vi "change channel raw default value.vi"(7 "owner ID":string, 8 "error in":errorcluster, 9 "raw default":string, 10 "channel name":string, 11 "engine configuration in":refnum<class "base TBM sequencer configuration.lvclass">) -> (0 "error out":errorcluster, 3 "engine configuration out":refnum<class "base TBM sequencer configuration.lvclass">)   [LabVIEW 2014, in "base TBM sequencer configuration.lvclass"]
uses:
  base TBM sequencer configuration.lvclass
  <vilib>/NI/Tag Bus/tag/tag descriptor.lvclass
  <vilib>/NI/Tag Bus/tag/tag descriptor.lvclass/tag descriptor.ctl
  base TBM sequencer configuration.lvclass/base TBM sequencer configuration.ctl
  <vilib>/NI/Tag Bus/tag/write tag name.vi
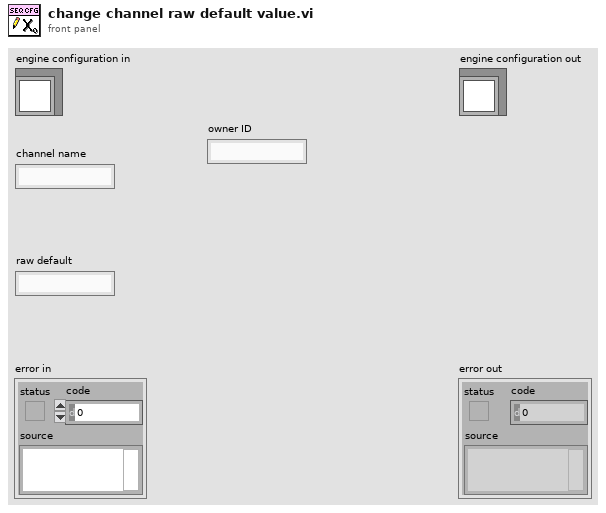
[diagram p1: front panel]
types:
  T1 = typedef "base TBM sequencer configuration.lvclass/Tag Info.ctl" = cluster{"Channel":refnum<class "TBM channel.lvclass">, "Writers":string[], "Readers":string[], "Owning ID":string}
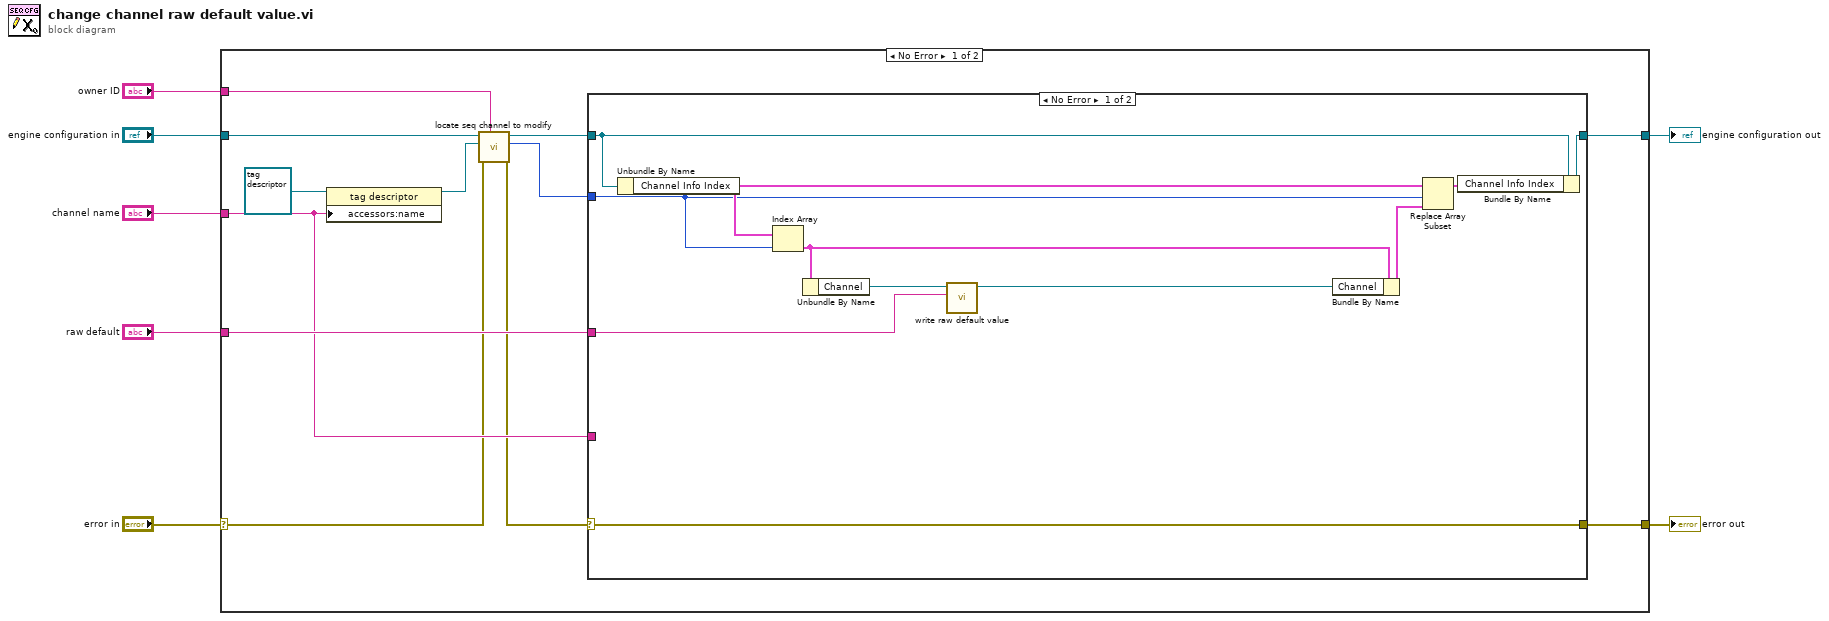
[diagram p0: block diagram]
diagram:
  n1 = case shown="No Error" "error in" {
    selector: "error in" -> [w10 w34]
    tunnel: [w17 w34] -> w6
    tunnel: [w18 w33] -> w4
    tunnel: "engine configuration in" -> [w14 w33]
    tunnel: "channel name" -> [w15 _]
    tunnel: "raw default" -> [w16 _]
    tunnel: "owner ID" -> [w11 _]
    frame No Error {
      n2 = property class="tag descriptor"(reference=refnum<class "tag descriptor.lvclass"> refnum ("tag descriptor"), "accessors:name"=w15) -> (reference out=w12:refnum<class "tag descriptor.lvclass">)  [unwired: 1 in, 1 out]
      n3 = call "locate seq channel to modify.vi"("owner ID"=w11, "error in"=w10, "tag descriptor"=w12, "engine configuration in"=w14) -> ("error out"=w9:errorcluster, "index"=w8:i32, "engine configuration out"=w13:refnum<class "base TBM sequencer configuration.lvclass">)  [unwired: 5 in]
      n4 = case shown="No Error" w9 {
        selector: w9 -> [w23 w31]
        tunnel: w13 -> [w25 w32]
        tunnel: [w26 w32] -> w18
        tunnel: [w23 w31] -> w17
        tunnel: w16 -> [w20 _]
        tunnel: w15 -> [_ _]
        tunnel: w8 -> [w24 _]
        frame No Error {
          n5 = Unbundle By Name(w25) -> ("Channel Info Index"=w29:T1[])
          n6 = Index Array(array=w29, index=w24) -> (element=w30:T1)
          n7 = Unbundle By Name(w30) -> ("Channel"=w22:refnum<class "TBM channel.lvclass">)
          n8 = call <vilib>:"write raw default value.vi"("raw default"=w20, "system tag in"=w22) -> ("system tag out"=w21:refnum<class "TBM channel.lvclass">)  [unwired: 8 in, 1 out]
          n9 = Bundle By Name(cluster=w30, "Channel"=w21) -> (w28:T1)
          n10 = Replace Array Subset(array=w29, new element=w28, index=w24) -> (w27:T1[])
          n11 = Bundle By Name(cluster=w25, "Channel Info Index"=w27) -> (w26:refnum<class "base TBM sequencer configuration.lvclass">)
        }
        frame Error {
        }
      }
    }
    frame Error {
    }
  }
  "error out" <- w6
  "engine configuration out" <- w4
